vi "GEA2 to HEUI.vi"(0 "HEUI_LEDs_In":T1, 13 "Raw Data In":string) -> (4 "HEUI_LEDs_Out":T1)   [LabVIEW 2016]
uses:
  Automation/Product Specific/Clothes Care/TL27/Product Testcode/VALEW/Valew Common/Display/controls/HEUI_LEDs.ctl
  Automation/Product Specific/Clothes Care/TL27/Projects/TL27.lvlib
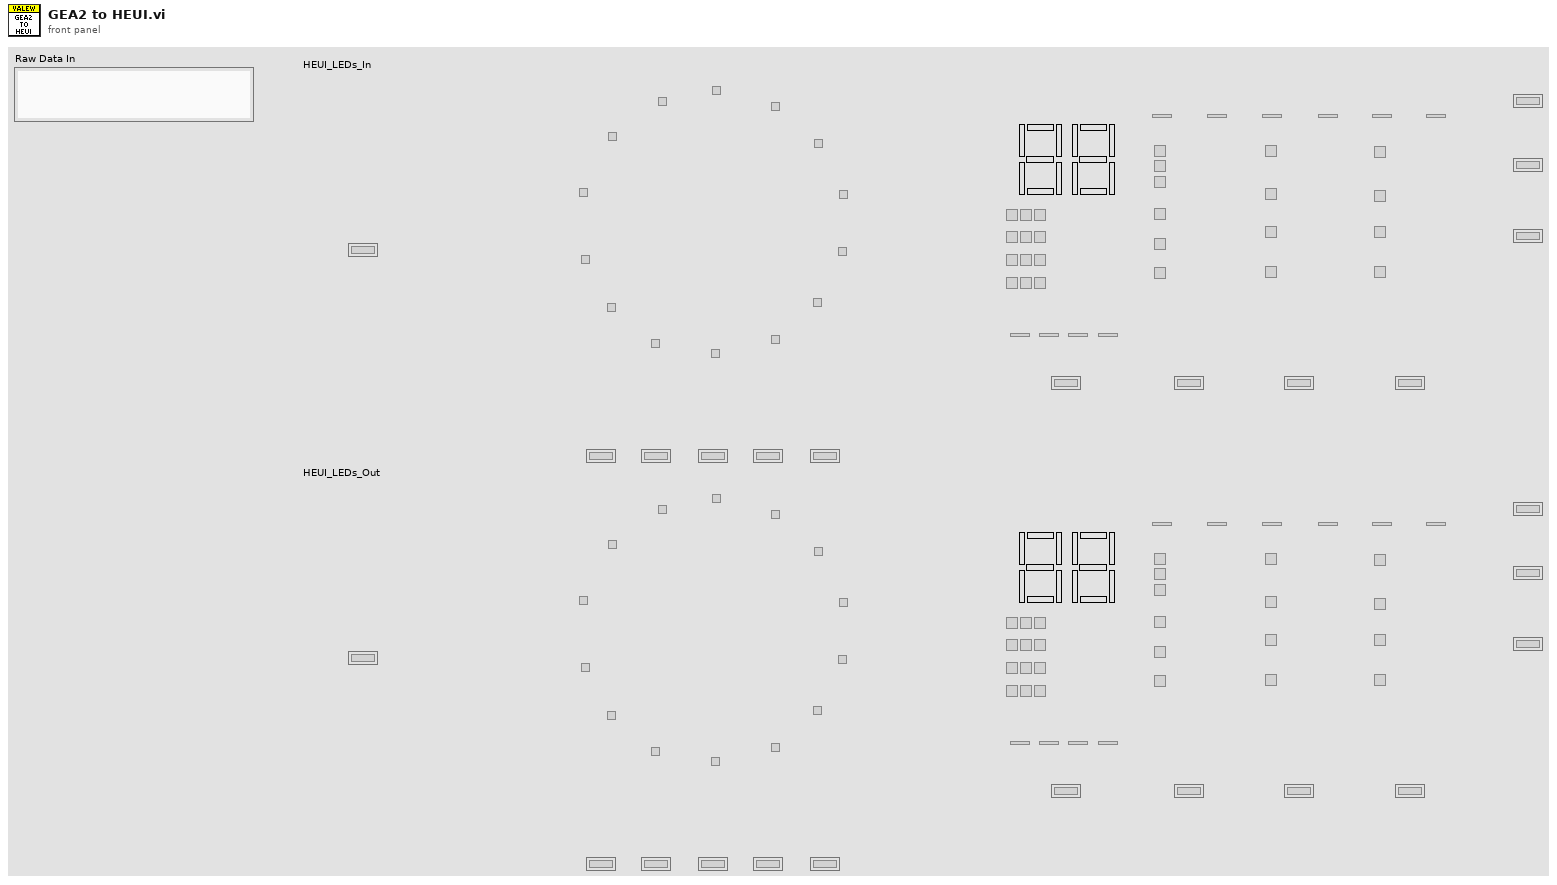
[diagram p1: front panel]
types:
  T1 = typedef "TL27.lvlib/HEUI_LEDs.ctl" = cluster{"Z101 - Start":bool, "Z103 - Colors":bool, "Z104 - Whites":bool, "Z105 - Towels":bool, "Z106 - Bulky Items":bool, "Z107 - Heavy Duty":bool, "Z108 - Jeans":bool, "Z109 - Basket Clean":bool, "Z110 - Drain and Spin":bool, "Z111 - Rinse and Spin":bool, "Z112 - Speed Wash":bool, "Z113 - Active Wear":bool, "Z114 - Hand Wash":bool, "Z115 - Delicates":bool, "Z116 - Easy Care":bool, "Z117 - Tomato":bool, "Z118 - Wine":bool, "Z119 - Blood":bool, "Z120 - Grass":bool, "Z121 - Dirt":bool, "Z122_MSB_A":bool, "Z123_MSB_B":bool, "Z124_MSB_G":bool, "Z125_MSB_C":bool, "Z126_MSB_D":bool, "Z127_MSB_E":bool, "Z128_MSB_F":bool, "Z129_LSB_A":bool, "Z130_LSB_B":bool, "Z131_LSB_G":bool, "Z132_LSB_C":bool, "Z133_LSB_D":bool, "Z134_LSB_E":bool, "Z135_LSB_F":bool, "Z136 - Pause":bool, "Z137 - Pause":bool, "Z138 - Lock Controls":bool, "Z139 - Lock Controls":bool, "Z140 - Lock Controls":bool, "Z141 - Lid Lock":bool, "Z142 - Lid Lock":bool, "Z143 - Lid Lock":bool, "Z144 - Good":bool, "Z145":bool, "Z146":bool, "Z147 - Better":bool, "Z148 - Delay":bool, "Z149 - Fill":bool, "Z150 - Soak":bool, "Z151 - Wash":bool, "Z152 - Rinse":bool, "Z153 - Spin":bool, "Z154 - Hot":bool, "Z155 - Warm":bool, "Z156 - Colors":bool, "Z157 - Cool":bool, "Z158 - Cold":bool, "Z159 - Tap Cold":bool, "Z160 - Extra Heavy":bool, "Z161 - Heavy":bool, "Z162 - Normal":bool, "Z163 - Light":bool, "Z164 - Max Spin":bool, "Z165 - More Spin":bool, "Z166 - Normal Spin":bool, "Z167 - No Spin":bool, "Z168 - Extra Rinse":bool, "Z170 - Deep Rinse":bool, "Z171 - Auto Soak":bool, "Z172 - Warm Rinse":bool, "Z173 - Deep Fill":bool, "Z174 - My Cycles":bool, "Z175 - Delay Wash":bool, "Z176 - Spin Stop":bool, "Z177 - Spin Stop":bool, "Z178 - Spin Stop":bool, "Z179 - Pause":bool, "Z109":bool, "Z110":bool, "Z123":bool, "Z124":bool, "Z140":bool, "Unused0":bool, "Unused1":bool, "Unused2":bool, "Unused3":bool, "Channel_Off":bool, "Channel_Cycle_Unmapped":bool}
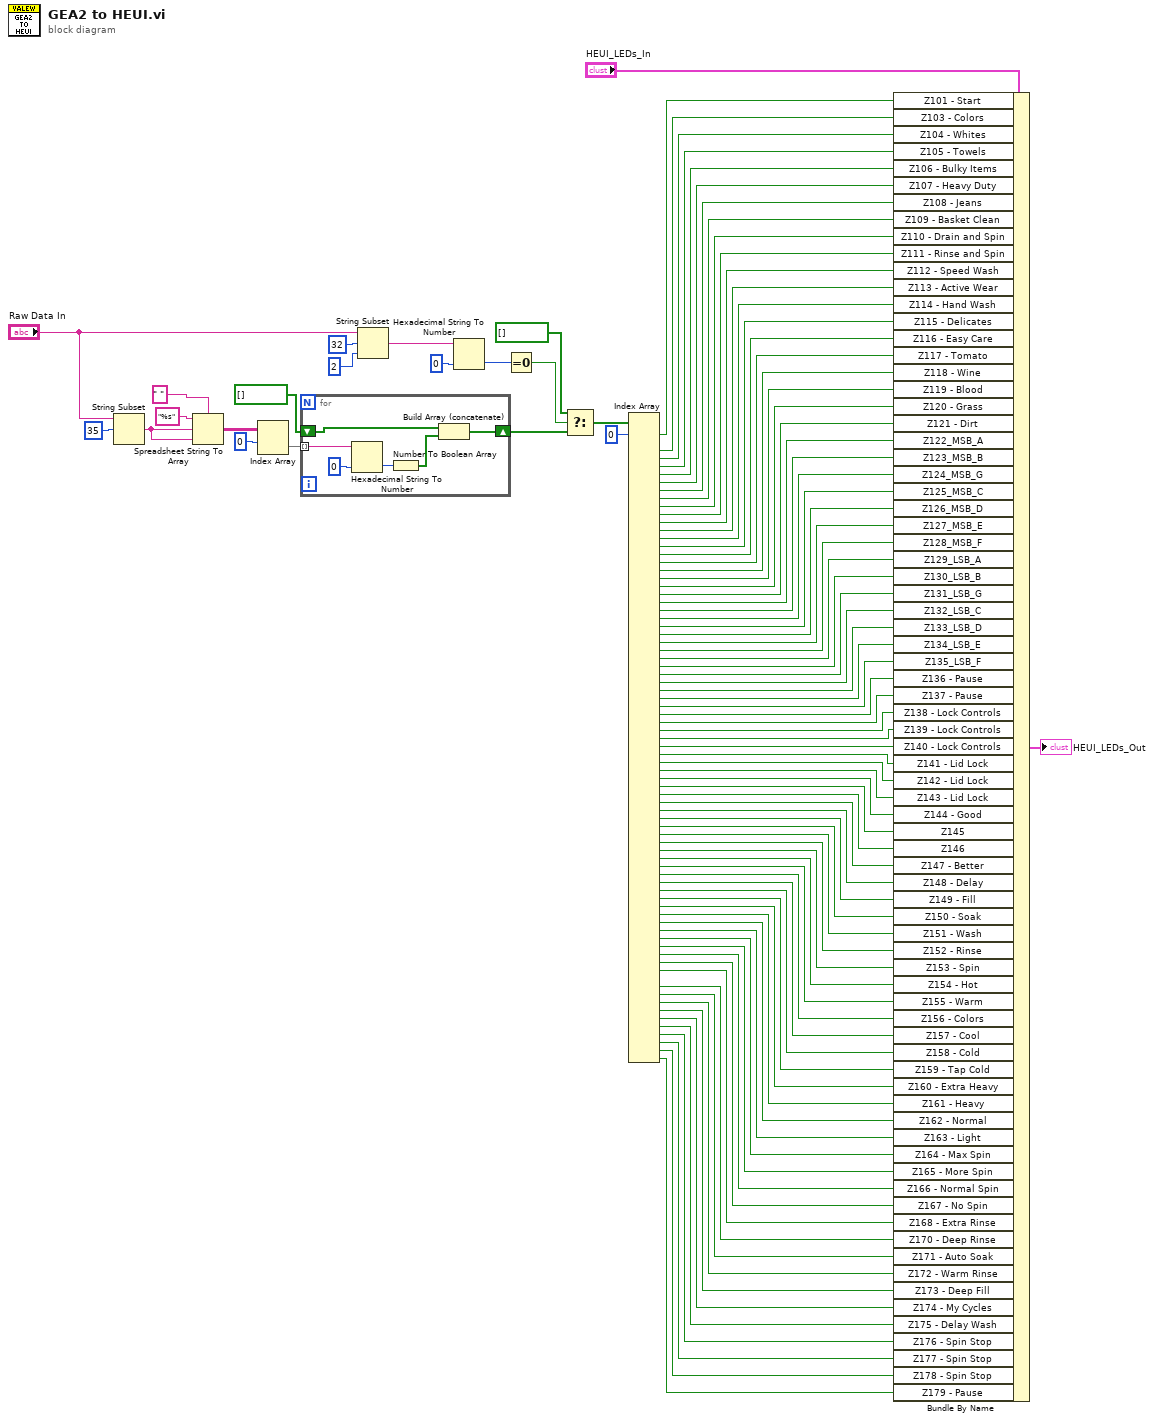
[diagram p0: block diagram]
diagram:
  n1 = String Subset(string="Raw Data In", offset (0)=35) -> (substring=w91:string)  [unwired: 1 in]
  n2 = Spreadsheet String To Array(delimiter (Tab)=" ", format string="%s", spreadsheet string=w91, array type (2D Dbl)=w91) -> (array=w95:string[][])
  n3 = Index Array(array=w95, index (row)=0) -> (element=w92:string[])  [unwired: 1 in]
  n4 = for {
    tunnel: w92 -> [w104] mode=indexing
    shift-right: [w100] -> w84
    shift-left: bool[] [] -> [w102]
    n5 = Hexadecimal String To Number(string=w104, default (0uL)=u8 0) -> (number=w103:u8)  [unwired: 1 in, 1 out]
    n6 = Number To Boolean Array(number=w103) -> (Boolean array=w101:bool[])
    n7 = Build Array (concatenate)(w102, w101) -> (w100:bool[])
  }
  n8 = String Subset(string="Raw Data In", offset (0)=32, length (rest)=2 ("length (rest)")) -> (substring=w88:string)
  n9 = Hexadecimal String To Number(string=w88, default (0uL)=u32 0 ("default (0 U32)")) -> (number=w86:u32)  [unwired: 1 in, 1 out]
  n10 = Equal To 0?(x=w86) -> (x = 0?=w85:bool)
  n11 = Select(t=bool[] [], s=w85, f=w84) -> (s? t:f=w82:bool[])
  n12 = Index Array(array=w82, index #1=0 ("index")) -> (element #1=w81:bool, element #3=w78:bool, element #4=w77:bool, element #5=w76:bool, element #6=w75:bool, element #7=w74:bool, element #8=w73:bool, element #9=w72:bool, element #10=w71:bool, element #11=w70:bool, element #12=w69:bool, element #13=w68:bool, element #14=w67:bool, element #15=w66:bool, element #16=w65:bool, element #17=w64:bool, element #18=w63:bool, element #19=w60:bool, element #20=w59:bool, element #21=w58:bool, element #22=w57:bool, element #23=w56:bool, element #24=w55:bool, element #25=w54:bool, element #26=w53:bool, element #27=w52:bool, element #28=w51:bool, element #29=w50:bool, element #30=w49:bool, element #31=w48:bool, element #32=w47:bool, element #33=w46:bool, element #34=w45:bool, element #35=w44:bool, element #36=w43:bool, element #37=w42:bool, element #38=w41:bool, element #39=w40:bool, element #40=w39:bool, element #41=w38:bool, element #42=w37:bool, element #43=w36:bool, element #44=w35:bool, element #45=w34:bool, element #46=w33:bool, element #47=w32:bool, element #48=w31:bool, element #49=w30:bool, element #50=w29:bool, element #51=w28:bool, element #52=w27:bool, element #53=w26:bool, element #54=w25:bool, element #55=w24:bool, element #56=w23:bool, element #57=w22:bool, element #58=w21:bool, element #59=w20:bool, element #60=w19:bool, element #61=w18:bool, element #62=w17:bool, element #63=w16:bool, element #64=w15:bool, element #65=w14:bool, element #66=w13:bool, element #67=w12:bool, element #68=w1:bool, element #70=w2:bool, element #71=w3:bool, element #72=w4:bool, element #73=w5:bool, element #74=w6:bool, element #75=w7:bool, element #76=w8:bool, element #77=w9:bool, element #78=w10:bool, element #79=w11:bool)  [unwired: 78 in, 2 out]
  n13 = Bundle By Name(cluster="HEUI_LEDs_In", "Z101 - Start"=w81, "Z103 - Colors"=w78, "Z104 - Whites"=w77, "Z105 - Towels"=w76, "Z106 - Bulky Items"=w75, "Z107 - Heavy Duty"=w74, "Z108 - Jeans"=w73, "Z109 - Basket Clean"=w72, "Z110 - Drain and Spin"=w71, "Z111 - Rinse and Spin"=w70, "Z112 - Speed Wash"=w69, "Z113 - Active Wear"=w68, "Z114 - Hand Wash"=w67, "Z115 - Delicates"=w66, "Z116 - Easy Care"=w65, "Z117 - Tomato"=w64, "Z118 - Wine"=w63, "Z119 - Blood"=w60, "Z120 - Grass"=w59, "Z121 - Dirt"=w58, "Z122_MSB_A"=w57, "Z123_MSB_B"=w56, "Z124_MSB_G"=w55, "Z125_MSB_C"=w54, "Z126_MSB_D"=w53, "Z127_MSB_E"=w52, "Z128_MSB_F"=w51, "Z129_LSB_A"=w50, "Z130_LSB_B"=w49, "Z131_LSB_G"=w48, "Z132_LSB_C"=w47, "Z133_LSB_D"=w46, "Z134_LSB_E"=w45, "Z135_LSB_F"=w44, "Z136 - Pause"=w43, "Z137 - Pause"=w42, "Z138 - Lock Controls"=w41, "Z139 - Lock Controls"=w40, "Z140 - Lock Controls"=w39, "Z141 - Lid Lock"=w38, "Z142 - Lid Lock"=w37, "Z143 - Lid Lock"=w36, "Z144 - Good"=w35, "Z145"=w34, "Z146"=w33, "Z147 - Better"=w32, "Z148 - Delay"=w31, "Z149 - Fill"=w30, "Z150 - Soak"=w29, "Z151 - Wash"=w28, "Z152 - Rinse"=w27, "Z153 - Spin"=w26, "Z154 - Hot"=w25, "Z155 - Warm"=w24, "Z156 - Colors"=w23, "Z157 - Cool"=w22, "Z158 - Cold"=w21, "Z159 - Tap Cold"=w20, "Z160 - Extra Heavy"=w19, "Z161 - Heavy"=w18, "Z162 - Normal"=w17, "Z163 - Light"=w16, "Z164 - Max Spin"=w15, "Z165 - More Spin"=w14, "Z166 - Normal Spin"=w13, "Z167 - No Spin"=w12, "Z168 - Extra Rinse"=w1, "Z170 - Deep Rinse"=w2, "Z171 - Auto Soak"=w3, "Z172 - Warm Rinse"=w4, "Z173 - Deep Fill"=w5, "Z174 - My Cycles"=w6, "Z175 - Delay Wash"=w7, "Z176 - Spin Stop"=w8, "Z177 - Spin Stop"=w9, "Z178 - Spin Stop"=w10, "Z179 - Pause"=w11) -> (→"HEUI_LEDs_Out":T1)
